vi "CoolSnap.vi"() -> ()   [LabVIEW 2012]
uses:
  <vilib>/Platform/TimedLoop/XDataNode/timing_clust.ctl
  <vilib>/Platform/TimedLoop/XDataNode/nitl_modes.ctl
  <vilib>/Platform/TimedLoop/XDataNode/wakeup.ctl
  <vilib>/Utility/error.llb/DialogType.ctl
  SITK/Documents/SIToolkit/LabVIEW/Examples2012_4_1_0_4/Open-Close/CamHandle.vi
  <vilib>/platform/TimedLoop/XDataNode/XDataNode.xnode
  <vilib>/Platform/TimedLoop/XDataNode/XDNodeRunTimeDep.lvlib
panel:
  in  "Tab Control":enum32{"Control", "Advanced"}(tab)
  in  "?":u16(ring) items=["Debug", "Bulb Trigger", "Free Run"]
  out "Image Monitor":i16[][](graph)
  in  "stop":bool
  in  "Number of Accumulations":u32=1
  in  "Number of Images":u32=1
  in  "Acquire / Focus Flag":u32(ring)=2 items=["Synchronous Focus Mode"=1, "Synchronous NFrame Mode"=2, "Asynchronous Mode"=3, "Sequence Mode"=4]
  in  "Errors":errorcluster
  in  "ADC Gain":i32=-1 min=-1 step=1
  in  "ADC Speed":i32=-1 min=-3 step=1
  in  "Exposure (sec)":dbl format="%.3f"
  in  "Timing Mode":u32(ring)=4 items=["Free Run"=1, "Trigger First"=2, "Strobe"=3, "Bulb"=4, "Variable"=5, "Flash"=6]
  in  "Trigger Edge":u32(ring)=1 items=["Rising"=1, "Falling"=2]
  in  "Camera Handle 2":u32
  in  "File and Display Name 2":string
  in  "error in (no error) 2":errorcluster
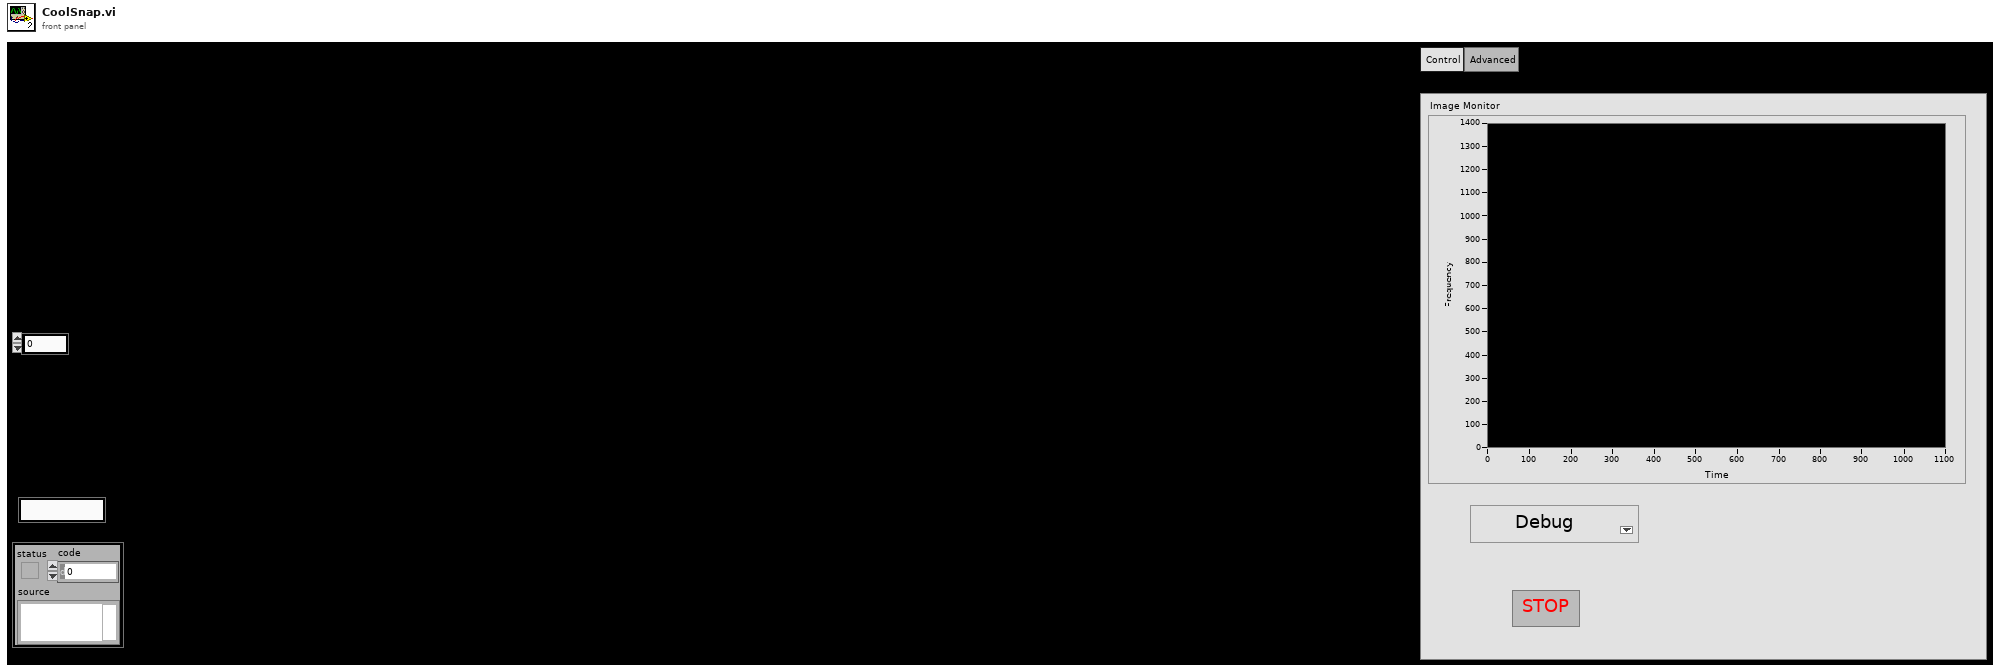
[diagram p1: front panel]
types:
  T1 = typedef "DialogType.ctl" = u16
  T2 = cluster{"Camera Handle":u32, "File Handle":u32, "Display Handle":u32, "Image Handle":u32}
  T3 = typedef "XDNodeRunTimeDep.lvlib/timing_clust.ctl" = cluster{"Expected End [f-1]":u64, "Actual End [f-1]":u64, "Finished Late? [f-1]":bool, "Expected End [i-1]":u64, "Actual End [i-1]":u64, "Finished Late? [i-1]":bool, "Expected Start [i]":u64, "Actual Start [i]":u64, "Expected Start [f]":u64, "Actual Start [f]":u64, "Source Name":string, "Structure Name":string, "Period":i64, "Deadline":i64, "Offset":i64, "Start":i64, "Priority":i32, "Timeout":i32, "Mode":T4, "Wakeup Reason":T5, "Error":errorcluster, "Source Type":string, "Secondary Source Type":string, "Global End Time":u64, "Global Start Time":u64, "Frame Duration":u64, "Iteration Duration":u64, "Assigned CPU":i32, "I/O Scan Engine Mode":u32}
  T4 = typedef "XDNodeRunTimeDep.lvlib/nitl_modes.ctl" = enum32{"No Change", "Process missed periods, maintain original phase", "Discard missed periods, maintain original phase", "Process missed periods, ignore original phase", "Discard missed periods, ignore original phase"}
  T5 = typedef "XDNodeRunTimeDep.lvlib/wakeup.ctl" = enum32{"Normal", "Aborted", "Asynchronous wakeup", "Timing source error", "Timed loop error", "Timeout"}
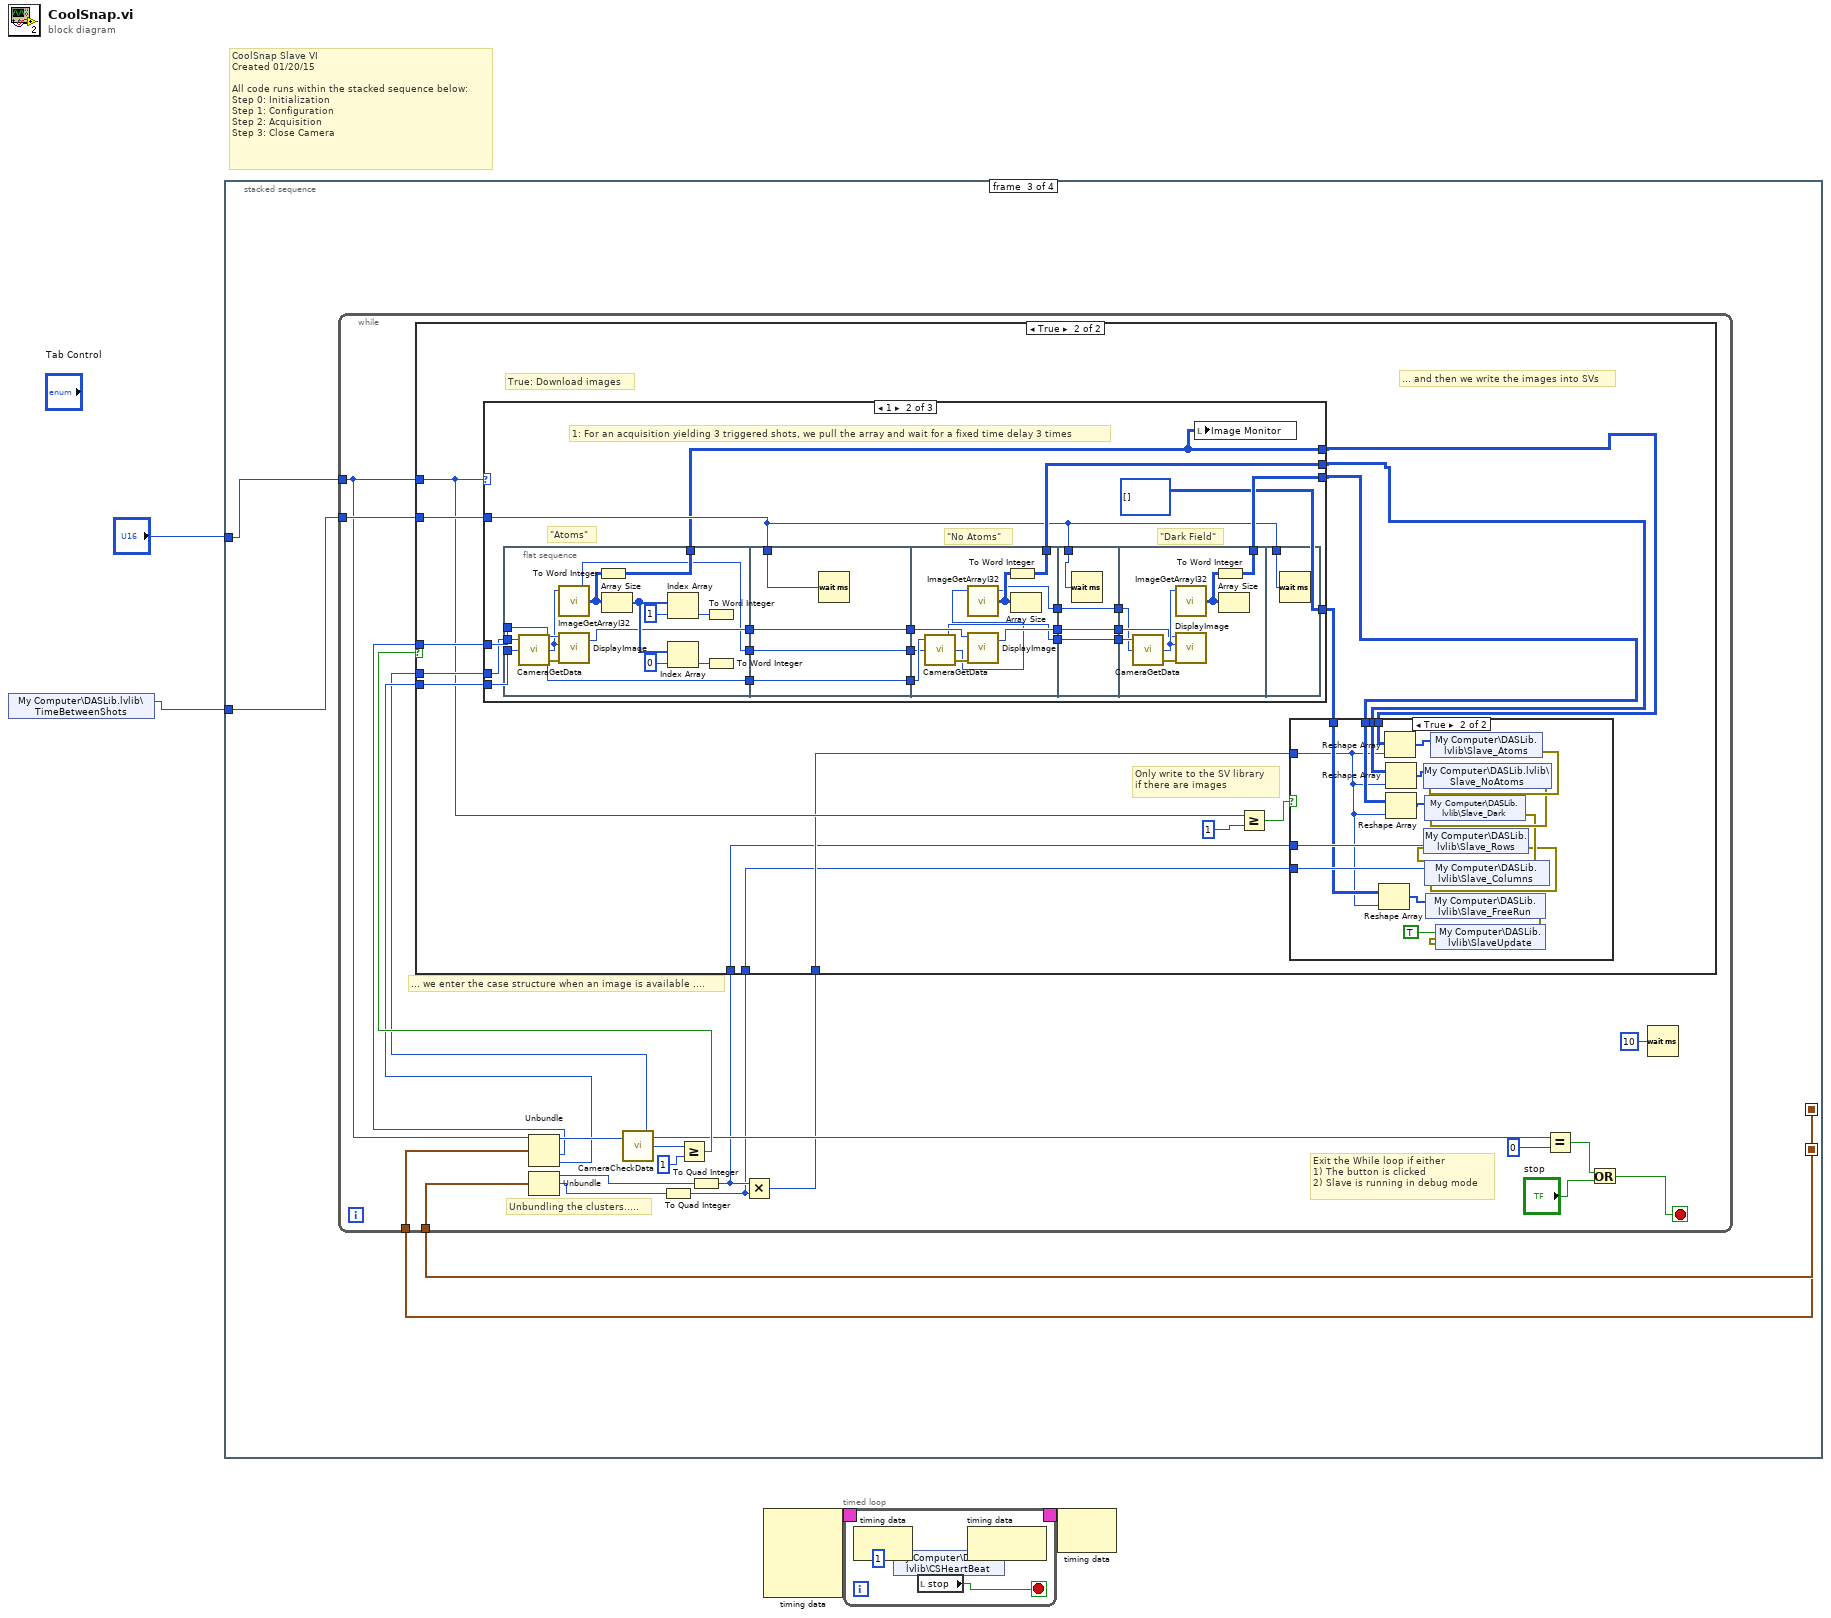
[diagram p0: block diagram]
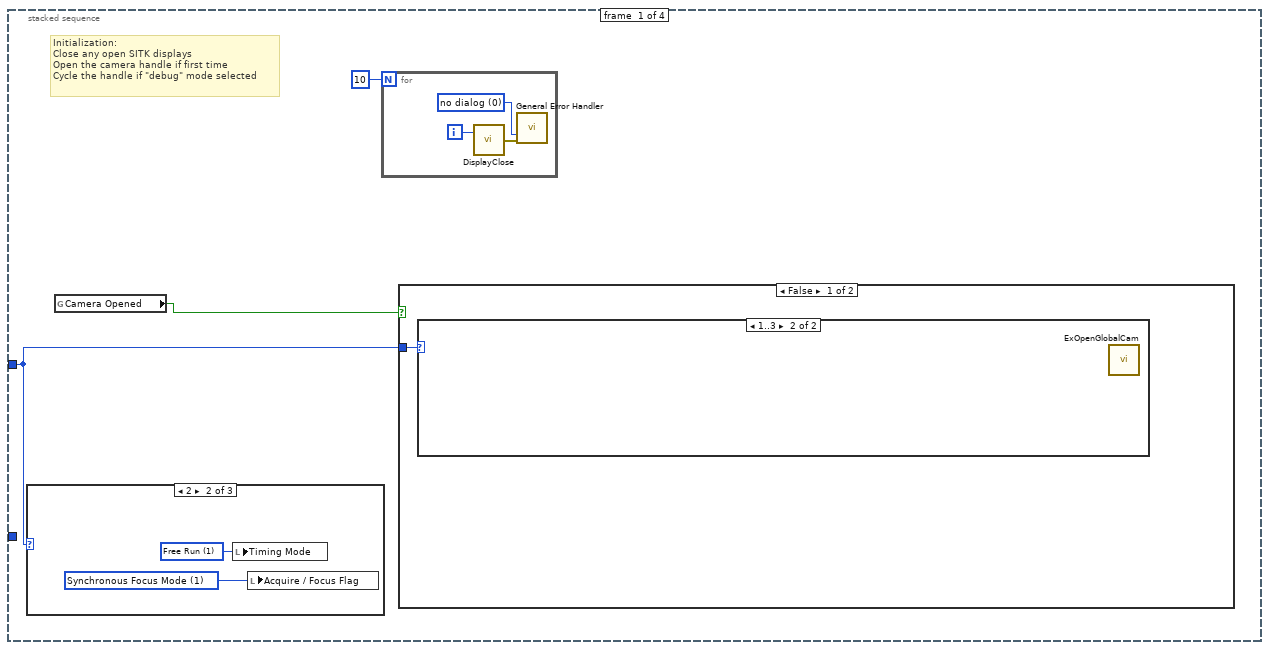
[diagram p2: hidden frame]
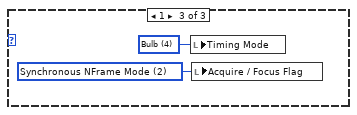
[diagram p4: hidden frame]
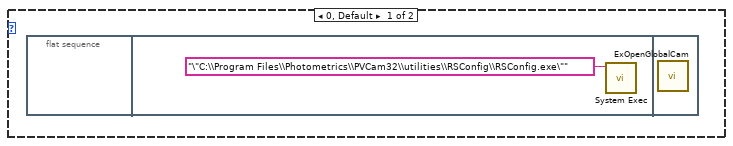
[diagram p5: hidden frame]
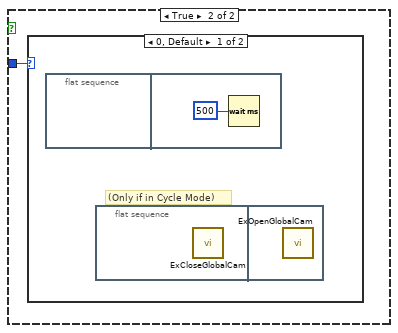
[diagram p6: hidden frame]
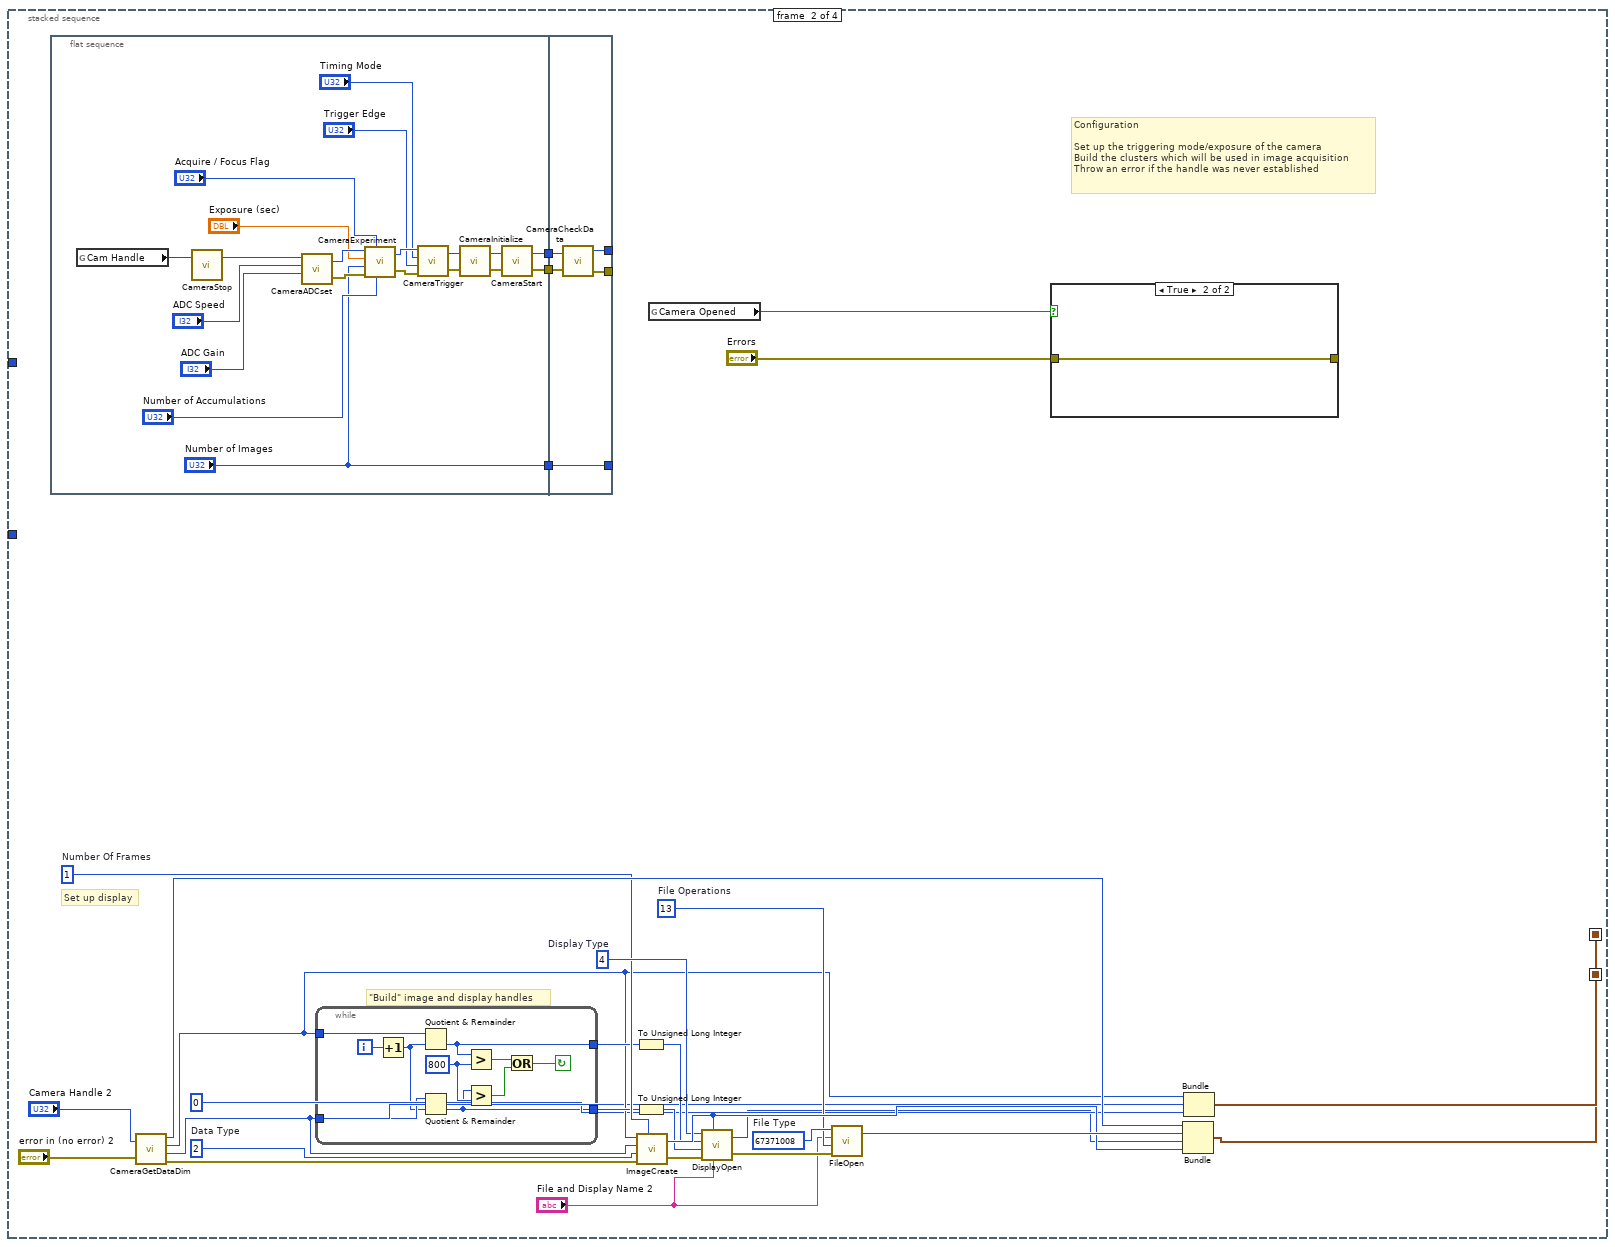
[diagram p8: hidden frame]
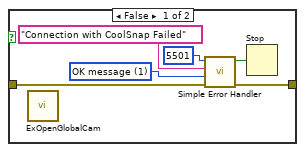
[diagram p9: hidden frame]
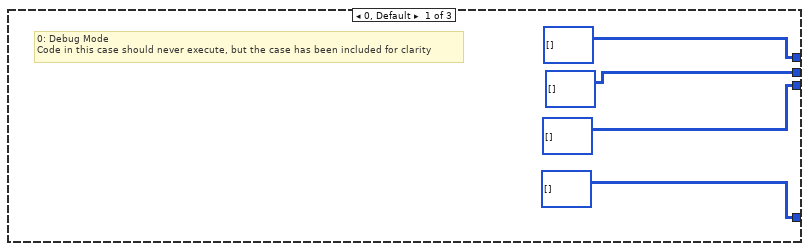
[diagram p12: hidden frame]
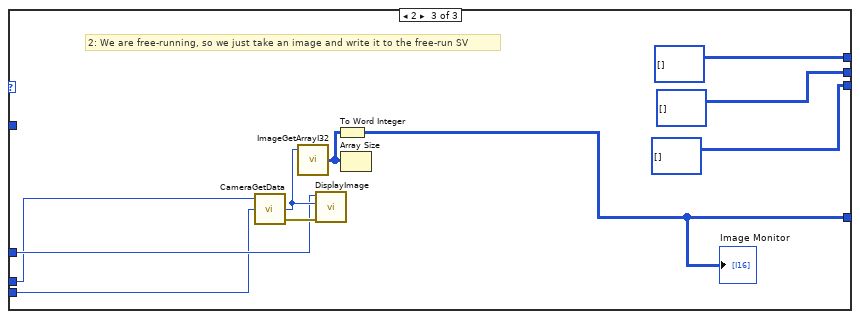
[diagram p13: hidden frame]
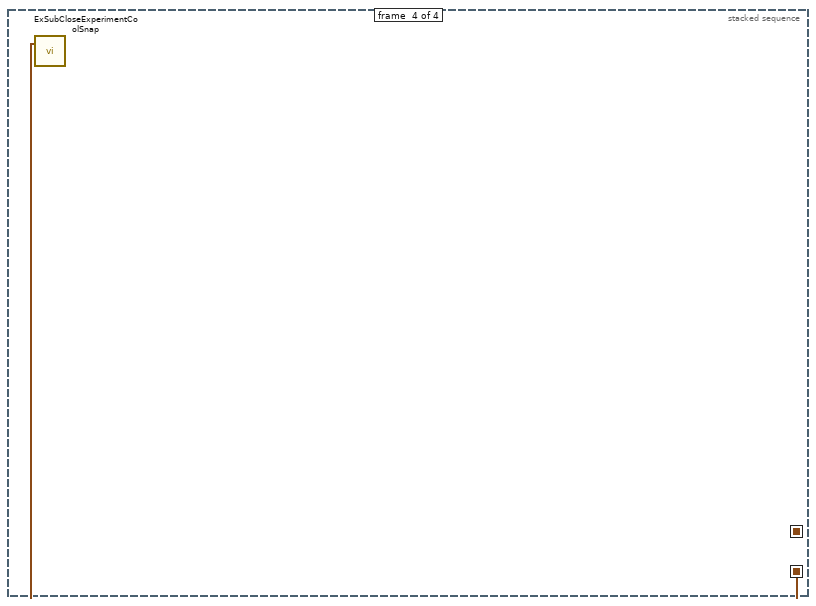
[diagram p14: hidden frame]
diagram:
  # "CoolSnap Slave VI\nCreated 01/20/15\n\nAll code runs within the stacked sequence below:\nStep 0: Initialization\nStep 1: Configuration\nStep 2: Acquisition\nStep 3: Close Camera"
  n1 = shared-variable "My Computer\\DASLib.lvlib\\TimeBetweenShots"() -> (w1:i64)  [unwired: 1 in, 1 out]
  n2 = stacked-sequence {
    seq-local: [_ w22 _ _] -> [_ _ w93 _]
    seq-local: [_ w21 _ _] -> [_ _ w90 w222]
    tunnel: "?" -> [w5 _ w92 _]
    tunnel: w1 -> [_ _ w91 _]
    frame #0 {
      # "Initialization:\nClose any open SITK displays\nOpen the camera handle if first time\nCycle the handle if \"debug\" mode selected"
      n3 = case shown="2" w5 {
        frame 0, Default {
        }
        frame 2 {
          w8 = u32 1 items=["Synchronous Focus Mode"=1, "Synchronous NFrame Mode"=2, "Asynchronous Mode"=3, "Sequence Mode"=4] ("Acquire / Focus Flag")
          w9 = u32 1 items=["Free Run"=1, "Trigger First"=2, "Strobe"=3, "Bulb"=4, "Variable"=5, "Flash"=6] ("Timing Mode")
          n4 = local write "Timing Mode"(w9) -> ()
          n5 = local write "Acquire / Focus Flag"(w8) -> ()
        }
        frame 1 {
          w10 = u32 2 items=["Synchronous Focus Mode"=1, "Synchronous NFrame Mode"=2, "Asynchronous Mode"=3, "Sequence Mode"=4] ("Acquire / Focus Flag")
          w11 = u32 4 items=["Free Run"=1, "Trigger First"=2, "Strobe"=3, "Bulb"=4, "Variable"=5, "Flash"=6] ("Timing Mode")
          n6 = local write "Timing Mode"(w11) -> ()
          n7 = local write "Acquire / Focus Flag"(w10) -> ()
        }
      }
      n8 = global read "CamHandle.vi" "Camera Opened"() -> (w6:bool)
      n9 = for {
        N: 10 -> [_]
        i -> [w18]
        w16 = T1 0 items=["no dialog", "OK message", "continue or stop message", "OK message + warnings", "continue/stop + warnings"] ("type of dialog (OK msg:1)")
        n10 = call <userlib>:"DisplayClose.vi"("Display Handle"=w18) -> ("error out"=w17:errorcluster)  [unwired: 1 in]
        n11 = call <vilib>:"General Error Handler.vi"("type of dialog (OK msg:1)"=w16, "error in (no error)"=w17) -> ()  [unwired: 9 in, 5 out]
      }
      n12 = case shown="False" w6 {
        tunnel: w5 -> [w12 w14]
        frame False {
          n13 = case shown="1..3" w12 {
            frame 0, Default {
              n14 = flat-sequence {
                frame #0 {
                }
                frame #1 {
                  n15 = call <vilib>:"System Exec.vi"("command line"="\"C:\\Program Files\\Photometrics\\PVCam32\\utilities\\RSConfig\\RSConfig.exe\"") -> ()  [unwired: 7 in, 4 out]
                }
                frame #2 {
                  n16 = call "ExOpenGlobalCam.vi"() -> ()  [unwired: 1 in]
                }
              }
            }
            frame 1..3 {
              n17 = call "ExOpenGlobalCam.vi"() -> ()  [unwired: 1 in]
            }
          }
        }
        frame True {
          n18 = case shown="0, Default" w14 {
            frame 0, Default {
              # "(Only if in Cycle Mode)"
              n19 = flat-sequence {
                frame #0 {
                }
                frame #1 {
                  n20 = Wait (ms)(milliseconds to wait=u32 500) -> ()  [unwired: 1 out]
                }
              }
              n21 = flat-sequence {
                frame #0 {
                  n22 = call "ExCloseGlobalCam.vi"() -> ()  [unwired: 1 in]
                }
                frame #1 {
                  n23 = call "ExOpenGlobalCam.vi"() -> ()  [unwired: 1 in]
                }
              }
            }
            frame 1..3 {
            }
          }
        }
      }
    }
    frame #1 {
      w31 = u32 1  # Number Of Frames
      w32 = u32 4  # Display Type
      w33 = u32 2  # Data Type
      w35 = 13  # File Operations
      w36 = 67371008  # File Type
      # "Configuration\n\nSet up the triggering mode/exposure of the camera\nBuild the clusters which will be used in image acquisition\nThrow an error if the handle was never established"
      # "\"Build\" image and display handles"
      # "Set up display"
      n24 = flat-sequence {
        tunnel: ["Number of Images"] -> w47
        tunnel: [w72] -> w46
        tunnel: [w71] -> w45
        tunnel: [w85] -> _
        tunnel: [w89] -> _
        tunnel: w47 -> [w89]
        tunnel: w46 -> [w88]
        tunnel: w45 -> [w87]
        tunnel: [w86] -> _
        frame #0 {
          n25 = global read "CamHandle.vi" "Cam Handle"() -> (w66:u32)
          n26 = call <userlib>:"CameraStop.vi"("Camera Handle"=w66) -> ("Camera Handle"=w67:u32)  [unwired: 1 in, 1 out]
          n27 = call <userlib>:"CameraADCset.vi"("ADC Gain"="ADC Gain", "ADC Speed"="ADC Speed", "Camera Handle"=w67) -> ("error out"=w82:errorcluster, "Camera Handle"=w84:u32)  [unwired: 3 in]
          n28 = call <userlib>:"CameraExperiment.vi"("Number of Accumulations"="Number of Accumulations", "Acquire / Focus Flag"="Acquire / Focus Flag", "error in"=w82, "Number of Images"="Number of Images", "Exposure (sec)"="Exposure (sec)", "Camera Handle"=w84) -> ("error out"=w76:errorcluster, "Camera Handle"=w77:u32)
          n29 = call <userlib>:"CameraTrigger.vi"("error in"=w76, "Trigger Edge"="Trigger Edge", "Timing Mode"="Timing Mode", "Camera Handle"=w77) -> ("error out"=w68:errorcluster, "Camera Handle"=w73:u32)
          n30 = call <userlib>:"CameraInitialize.vi"("error in"=w68, "Camera Handle"=w73) -> ("error out"=w70:errorcluster, "Camera Handle"=w69:u32)
          n31 = call <userlib>:"CameraStart.vi"("error in"=w70, "Camera Handle"=w69) -> ("error out"=w71:errorcluster, "Camera Handle"=w72:u32)
        }
        frame #1 {
          n32 = call <userlib>:"CameraCheckData.vi"("Camera Handle"=w88, "error in"=w87) -> ("Camera Handle"=w85:u32, "error out"=w86:errorcluster)  [unwired: 1 out]
        }
      }
      n33 = call <userlib>:"CameraGetDataDim.vi"("Camera Handle"="Camera Handle 2", "error in"="error in (no error) 2") -> ("Camera Handle"=w39:u32, "Xdim"=w26:u32, "Ydim"=w25:u32, "error out"=w44:errorcluster)
      n34 = while {
        tunnel: w26 -> [w63]
        tunnel: w25 -> [w62]
        tunnel: [w57] -> w30
        tunnel: [w56] -> w29
        i -> [w61]
        stop <- w58 continue-if-true
        w64 = 800
        n35 = Increment(x=w61) -> (x+1=w55:i32)
        n36 = Quotient & Remainder(x=w63, y=w55) -> (floor(x/y)=w57:u32)  [unwired: 1 out]
        n37 = Quotient & Remainder(x=w62, y=w55) -> (floor(x/y)=w56:u32)  [unwired: 1 out]
        n38 = Greater?(x=w57, y=w64) -> (0:w60:bool)
        n39 = Greater?(x=w56, y=w64) -> (0:w59:bool)
        n40 = Or(x=w60, y=w59) -> (x .or. y?=w58:bool)
      }
      n41 = To Unsigned Long Integer(number=w30) -> (unsigned 32bit integer=w28:u32)
      n42 = To Unsigned Long Integer(number=w29) -> (unsigned 32bit integer=w27:u32)
      n43 = call <userlib>:"ImageCreate.vi"("X dimension"=w26, "Y dimension"=w25, "Data Type"=w33, "error in"=w44, "Number Of Frames"=w31) -> ("Image Handle"=w37:u32, "error out"=w43:errorcluster)
      n44 = global read "CamHandle.vi" "Camera Opened"() -> (w20:bool)
      n45 = call <userlib>:"DisplayOpen.vi"("Display Title"="File and Display Name 2", "Image Handle"=w37, "error in"=w43, "Display Height"=w27, "Display Width"=w28, "Display Type"=w32) -> ("error out"=w42:errorcluster, "Display Handle"=w23:u32)
      n46 = call <userlib>:"FileOpen.vi"("error in"=w42, "File Operations"=w35, "FileName"="File and Display Name 2", "File Type"=w36) -> ("File Handle"=w38:u32)  [unwired: 1 out]
      n47 = case shown="True" w20 {
        tunnel: [w52 w54] -> _
        tunnel: "Errors" -> [w48 w54]
        frame False {
          w53 = u16 1 items=["no dialog", "OK message", "continue or stop message"] ("type of dialog (OK msg:1)")
          n48 = call "ExOpenGlobalCam.vi"() -> ()  [unwired: 1 in]
          n49 = call <vilib>:"Simple Error Handler.vi"("error code (no error:0)"=5501, "error source (\" \")"="Connection with CoolSnap Failed", "type of dialog (OK msg:1)"=w53, "error in (no error)"=w48) -> ("error?"=w50:bool, "error out"=w52:errorcluster)  [unwired: 1 in, 3 out]
          n50 = Stop(stop? (T)=w50) -> ()
        }
        frame True {
        }
      }
      n51 = Bundle("Camera Handle"=w39, "File Handle"=w38, "Display Handle"=w23, "Image Handle"=w37) -> (w21:T2)  [unwired: 1 in]
      n52 = Bundle("Xdim"=w26, "Ydim"=w25, 0) -> (w22:cluster{"Xdim":u32, "Ydim":u32, i32})  [unwired: 1 in]
    }
    frame #2 {
      n53 = while {
        tunnel: w93 -> [w114]
        tunnel: w90 -> [w113]
        tunnel: w92 -> [w100]
        tunnel: w91 -> [w101]
        stop <- w103 stop-if-true
        # "... we enter the case structure when an image is available ...."
        # "Unbundling the clusters....."
        # "Exit the While loop if either\n1) The button is clicked\n2) Slave is running in debug mode"
        n54 = Unbundle(w113) -> ("Camera Handle"=w112:u32, "Display Handle"=w107:u32, "Image Handle"=w108:u32)  [unwired: 1 out]
        n55 = Unbundle(w114) -> ("Xdim"=w98:u32, "Ydim"=w97:u32)  [unwired: 1 out]
        n56 = call <userlib>:"CameraCheckData.vi"("Camera Handle"=w112) -> ("Camera Handle"=w106:u32, "Number Of Frames Available"=w111:i32)  [unwired: 1 in, 1 out]
        n57 = To Quad Integer(1:w97) -> (0:w94:i64)
        n58 = Greater Or Equal?(x=w111, y=1) -> (x >= y?=w109:bool)
        n59 = To Quad Integer(1:w98) -> (0:w95:i64)
        n60 = Multiply(x=w95, y=w94) -> (x*y=w99:i64)
        n61 = case shown="True" w109 {
          tunnel: w106 -> [_ w127]
          tunnel: w108 -> [_ w126]
          tunnel: w107 -> [_ w128]
          tunnel: w100 -> [_ w122]
          tunnel: w101 -> [_ w125]
          tunnel: w99 -> [_ w121]
          tunnel: w95 -> [_ w120]
          tunnel: w94 -> [_ w119]
          frame False {
            # "False: Keep waiting for images"
          }
          frame True {
            # "Only write to the SV library \nif there are images"
            # "... and then we write the images into SVs"
            # "True: Download images"
            n62 = case shown="1" w122 {
              tunnel: w128 -> [_ w170 w218]
              tunnel: w127 -> [_ w169 w217]
              tunnel: w126 -> [_ w168 w216]
              tunnel: w125 -> [_ w157 _]
              tunnel: [i16[][] [] w155 i16[][] []] -> w118
              tunnel: [i16[][] [] w159 i16[][] []] -> w117
              tunnel: [i16[][] [] w158 i16[][] []] -> w116
              tunnel: [i16[][] [] i16[][] [] w212] -> w115
              frame 0, Default {
                # "0: Debug Mode\nCode in this case should never execute, but the case has been included for clarity"
              }
              frame 1 {
                # "\"Dark Field\""
                # "\"No Atoms\""
                # "\"Atoms\""
                # "1: For an acquisition yielding 3 triggered shots, we pull the array and wait for a fixed time delay 3 times"
                n63 = flat-sequence {
                  tunnel: w170 -> [w185]
                  tunnel: w169 -> [w184]
                  tunnel: w168 -> [w183]
                  tunnel: [w175] -> w166
                  tunnel: [w173] -> w161
                  tunnel: [w174] -> w155
                  tunnel: [w172] -> w154
                  tunnel: w157 -> [w189]
                  tunnel: [w188] -> w167
                  tunnel: w166 -> [w188]
                  tunnel: w161 -> [w187]
                  tunnel: [w187] -> w160
                  tunnel: w154 -> [w186]
                  tunnel: [w186] -> w153
                  tunnel: w167 -> [w197]
                  tunnel: [w196] -> w164
                  tunnel: [w195] -> w163
                  tunnel: w160 -> [w194]
                  tunnel: [w193] -> w159
                  tunnel: w153 -> [w191]
                  tunnel: [w190] -> w151
                  tunnel: [w203] -> w165
                  tunnel: w164 -> [w203]
                  tunnel: w163 -> [w202]
                  tunnel: [w202] -> w162
                  tunnel: w157 -> [w201]
                  tunnel: [w200] -> w152
                  tunnel: w151 -> [w200]
                  tunnel: w165 -> [w207]
                  tunnel: w162 -> [w206]
                  tunnel: [w205] -> w158
                  tunnel: w152 -> [w204]
                  tunnel: w157 -> [w211]
                  frame #0 {
                    n64 = call <userlib>:"CameraGetData.vi"("Data Handle"=w183, "Camera Handle"=w184) -> ("error out"=w182:errorcluster, "Data Handle"=w171:u32, "Camera Handle"=w173:u32)  [unwired: 1 in]
                    n65 = call <userlib>:"ImageGetArrayI32.vi"("Image Handle"=w171) -> ("Array int 32"=w176:i32[][], "Image Handle"=w172:u32)  [unwired: 2 in, 1 out]
                    n66 = call <userlib>:"DisplayImage.vi"("error in"=w182, "Image Handle"=w171, "Display Handle"=w185) -> ("Display Handle"=w175:u32)  [unwired: 1 in, 1 out]
                    n67 = To Word Integer(number=w176) -> (16bit integer=w174:i16[][])
                    n68 = Array Size(array=w176) -> (size(s)=w177:i32[])
                    n69 = Index Array(array=w177, index=1) -> (element=w178:i32)
                    n70 = Index Array(array=w177, index=0) -> (element=w179:i32)
                    n71 = To Word Integer(number=w178) -> ()  [unwired: 1 out]
                    n72 = To Word Integer(number=w179) -> ()  [unwired: 1 out]
                  }
                  frame #1 {
                    n73 = Wait (ms)(milliseconds to wait=w189) -> ()  [unwired: 1 out]
                  }
                  frame #2 {
                    n74 = call <userlib>:"CameraGetData.vi"("Data Handle"=w191, "Camera Handle"=w194) -> ("error out"=w199:errorcluster, "Data Handle"=w192:u32, "Camera Handle"=w195:u32)  [unwired: 1 in]
                    n75 = call <userlib>:"ImageGetArrayI32.vi"("Image Handle"=w192) -> ("Array int 32"=w198:i32[][], "Image Handle"=w190:u32)  [unwired: 2 in, 1 out]
                    n76 = call <userlib>:"DisplayImage.vi"("error in"=w199, "Display Handle"=w197) -> ("Display Handle"=w196:u32)  [unwired: 2 in, 1 out]
                    n77 = To Word Integer(number=w198) -> (16bit integer=w193:i16[][])
                    n78 = Array Size(array=w198) -> ()  [unwired: 1 out]
                  }
                  frame #3 {
                    n79 = Wait (ms)(milliseconds to wait=w201) -> ()  [unwired: 1 out]
                  }
                  frame #4 {
                    n80 = call <userlib>:"CameraGetData.vi"("Data Handle"=w204, "Camera Handle"=w206) -> ("error out"=w210:errorcluster, "Data Handle"=w209:u32)  [unwired: 1 in, 1 out]
                    n81 = call <userlib>:"ImageGetArrayI32.vi"("Image Handle"=w209) -> ("Array int 32"=w208:i32[][])  [unwired: 2 in, 2 out]
                    n82 = call <userlib>:"DisplayImage.vi"("error in"=w210, "Image Handle"=w209, "Display Handle"=w207) -> ()  [unwired: 1 in, 2 out]
                    n83 = To Word Integer(number=w208) -> (16bit integer=w205:i16[][])
                    n84 = Array Size(array=w208) -> ()  [unwired: 1 out]
                  }
                  frame #5 {
                    n85 = Wait (ms)(milliseconds to wait=w211) -> ()  [unwired: 1 out]
                  }
                }
                n86 = local write "Image Monitor"(w155) -> ()
              }
              frame 2 {
                # "2: We are free-running, so we just take an image and write it to the free-run SV"
                n87 = call <userlib>:"CameraGetData.vi"("Data Handle"=w216, "Camera Handle"=w217) -> ("error out"=w221:errorcluster, "Data Handle"=w220:u32)  [unwired: 1 in, 1 out]
                n88 = call <userlib>:"ImageGetArrayI32.vi"("Image Handle"=w220) -> ("Array int 32"=w219:i32[][])  [unwired: 2 in, 2 out]
                n89 = call <userlib>:"DisplayImage.vi"("error in"=w221, "Image Handle"=w220, "Display Handle"=w218) -> ()  [unwired: 1 in, 2 out]
                n90 = To Word Integer(number=w219) -> (16bit integer=w212:i16[][])
                "Image Monitor" <- w212
                n91 = Array Size(array=w219) -> ()  [unwired: 1 out]
              }
            }
            n92 = Greater Or Equal?(x=w122, y=1 ("index")) -> (x >= y?=w123:bool)
            n93 = case shown="True" w123 {
              tunnel: w117 -> [_ w146]
              tunnel: w118 -> [_ w145]
              tunnel: w116 -> [_ w144]
              tunnel: w121 -> [_ w136]
              tunnel: w120 -> [_ w140]
              tunnel: w119 -> [_ w139]
              tunnel: w115 -> [_ w137]
              frame False {
                # "No bombarding the SV library with free-run\nimages!"
              }
              frame True {
                n94 = Reshape Array(w137, w136) -> (w138:i16[])
                n95 = Reshape Array(w145, w136) -> (w143:i16[])
                n96 = Reshape Array(w146, w136) -> (w142:i16[])
                n97 = Reshape Array(w144, w136) -> (w141:i16[])
                n98 = shared-variable "My Computer\\DASLib.lvlib\\Slave_Atoms"(w143) -> (error out=w133:errorcluster)  [unwired: 1 in]
                n99 = shared-variable "My Computer\\DASLib.lvlib\\Slave_NoAtoms"(w142, error in=w133) -> (error out=w132:errorcluster)
                n100 = shared-variable "My Computer\\DASLib.lvlib\\Slave_Dark"(w141, error in=w132) -> (error out=w131:errorcluster)
                n101 = shared-variable "My Computer\\DASLib.lvlib\\Slave_Rows"(w140, error in=w131) -> (error out=w130:errorcluster)
                n102 = shared-variable "My Computer\\DASLib.lvlib\\Slave_Columns"(w139, error in=w130) -> (error out=w129:errorcluster)
                n103 = shared-variable "My Computer\\DASLib.lvlib\\Slave_FreeRun"(w138, error in=w129) -> (error out=w135:errorcluster)
                n104 = shared-variable "My Computer\\DASLib.lvlib\\SlaveUpdate"(TRUE ("SlaveUpdate"), error in=w135) -> ()  [unwired: 1 out]
              }
            }
          }
        }
        n105 = Equal?(x=w100, y=0 ("index")) -> (x = y?=w104:bool)
        n106 = Or(x=w104, y="stop") -> (x .or. y?=w103:bool)
        n107 = Wait (ms)(milliseconds to wait=u32 10) -> ()  [unwired: 1 out]
      }
    }
    frame #3 {
      n108 = call "ExSubCloseExperimentCoolSnap.vi"("Handles In"=w222) -> ()  [unwired: 1 in, 1 out]
    }
  }
  n109 = node-c288() -> (w3:T3)  [unwired: 4 in]
  n110 = timed-loop {
    timing: w3 -> [_]
    timing-out: [_] -> w2
    stop <- w223 stop-if-true
    n111 = node-c288() -> ()  [unwired: 1 in, 1 out]
    n112 = shared-variable "My Computer\\DASLib.lvlib\\CSHeartBeat"(i16 1 ("PFHeartBeat")) -> ()  [unwired: 1 in, 1 out]
    n113 = local read "stop"() -> (w223:bool)
    n114 = node-c288() -> ()  [unwired: 1 in, 1 out]
  }
  n115 = node-c288(w2) -> ()  [unwired: 1 out]
